vi "getY2Corr.vi"(8 "error in (no error)":errorcluster, 10 "Field Idx":i32[](array[numeric]), 11 "OptStateEsti in":refnum<class "OptStateEsti.lvclass">) -> (0 "error out":errorcluster, 2 "y2c Array":dbl[][](array[numeric]), 3 "OptStateEsti out":refnum<class "OptStateEsti.lvclass">)   [LabVIEW 2016, in "OptStateEsti.lvclass"]
doc: "Get the y2 correction array in nx1 shape."
uses:
  OptStateEsti.lvclass
  OptStateEsti.lvclass/OptStateEsti.ctl
panel:
  in  "y2 Corection File Name":string="y2.txt"
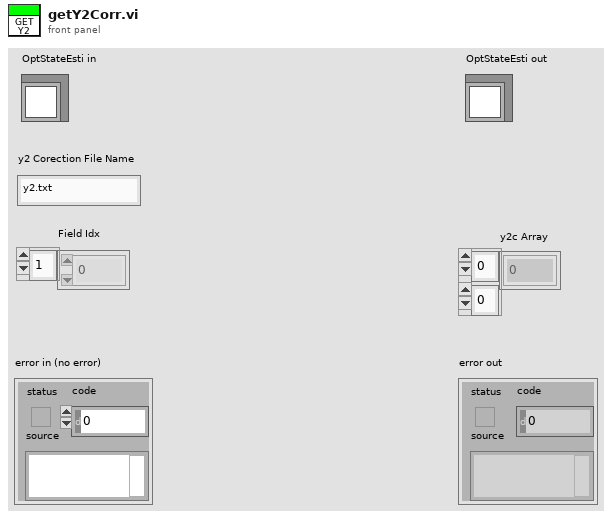
[diagram p1: front panel]
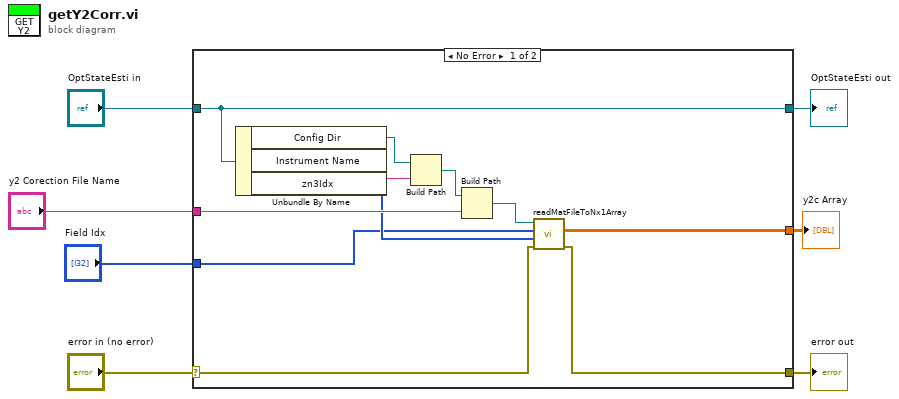
[diagram p0: block diagram]
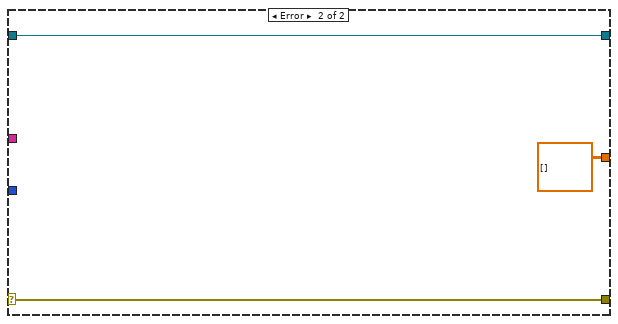
[diagram p2: hidden frame]
diagram:
  n1 = case shown="No Error" "error in (no error)" {
    selector: "error in (no error)" -> [w12 w21]
    tunnel: [w11 w21] -> w6
    tunnel: [w18 w20] -> w4
    tunnel: "OptStateEsti in" -> [w18 w20]
    tunnel: "y2 Corection File Name" -> [w14 _]
    tunnel: [w10 dbl[][] [] ("nx1 Array")] -> w2
    tunnel: "Field Idx" -> [w8 _]
    frame No Error {
      n2 = Unbundle By Name(w18) -> ("Config Dir"=w17:path, "Instrument Name"=w16:string, "zn3Idx"=w9:i32[])
      n3 = Build Path(base path=w17, name or relative path=w16) -> (appended path=w15:path)
      n4 = Build Path(base path=w15, name or relative path=w14) -> (appended path=w13:path)
      n5 = call "readMatFileToNx1Array.vi"("error in (no error)"=w12, "Index of Column"=w9, "Index of Row"=w8, "Path"=w13) -> ("error out"=w11:errorcluster, "nx1 Array"=w10:dbl[][])  [unwired: 6 in]
    }
    frame Error {
    }
  }
  "error out" <- w6
  "OptStateEsti out" <- w4
  "y2c Array" <- w2
